vi "description.set.vi"(8 "error in (no error)":errorcluster, 10 "description":string, 11 "type in":refnum<class "type.lvclass">) -> (0 "error out":errorcluster, 3 "type out":refnum<class "type.lvclass">)   [LabVIEW 2020, in "type.lvclass"]
uses:
  type.lvclass
  type.lvclass/type.ctl
  Nominal Client/Nominal Client.lvclass
  f25efd28-d0c3-44dc-9fcd-1669f60030d2.vi
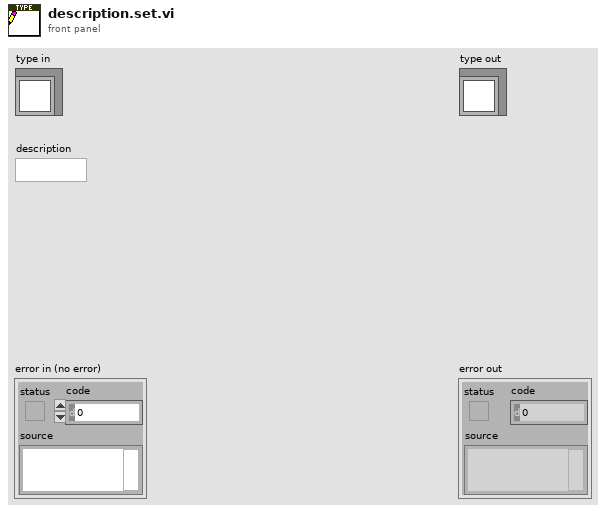
[diagram p1: front panel]
types:
  T1 = typedef "type.lvclass/typeData.ctl" = cluster{"rid":string, "name":string, "description":string, "propertyConfigs":T2, "createdAt":timestamp, "datasourceConfigs":T5[], "iconName":string}
  T2 = typedef "type.lvclass/properties.ctl" = T3[]
  T3 = typedef "type.lvclass/property.ctl" = cluster{"name":string, "value":T4}
  T4 = typedef "type.lvclass/property value.ctl" = cluster{"isRequired":bool, "description":string}
  T5 = typedef "type.lvclass/datasourceConfig.ctl" = cluster{"name":string, "v1":string[], "suggestedRefName":string}
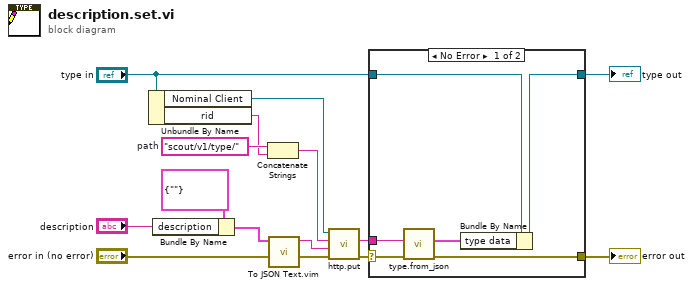
[diagram p0: block diagram]
diagram:
  w11 = "scout/v1/type/"  # path
  n1 = Unbundle By Name("type in") -> ("Nominal Client"=w15:refnum<class "Nominal Client.lvclass">, "rid"=w8:string)
  n2 = Bundle By Name(cluster=cluster{"description":string} {"description"=""}, "description"="description") -> (w13:cluster{"description":string})
  n3 = Concatenate Strings(w11, w8) -> (w10:string)
  n4 = call "To JSON Text.vim"("error in (no error)"="error in (no error)", "Anything"=w13) -> ("error out"=w9:errorcluster, "<JSON>"=w12:string)  [unwired: 8 in]
  n5 = call "http.put.vi"("error in"=w9, "Body"=w12, "Path"=w10, "Nominal Client in"=w15) -> ("error out"=w7:errorcluster, "Response"=w6:string)  [unwired: 4 in, 2 out]
  n6 = case shown="No Error" w7 {
    selector: w7 -> [w19 w23]
    tunnel: [w18 w23] -> w1
    tunnel: "type in" -> [w21 w22]
    tunnel: w6 -> [w17 _]
    tunnel: [w20 w22] -> w2
    frame No Error {
      n7 = call "type.from_json.vi"("error in"=w19, "json"=w17) -> ("error out"=w18:errorcluster, "type data"=w16:T1)  [unwired: 8 in]
      n8 = Bundle By Name(cluster=w21, "type data"=w16) -> (w20:refnum<class "type.lvclass">)
    }
    frame Error {
    }
  }
  "error out" <- w1
  "type out" <- w2
